vi "Configure Signaling RF UL Location A.vi"(8 "error in (no error)":errorcluster, 9 "UL Location A (Mid)":i32(ring) items=["Mid", "Low", "High", "User"], 10 "Cell Name (\"Cell Name\")":string="Cell Name", 11 "VISA resource name":refnum<visa-resource-name>) -> (0 "error out":errorcluster, 3 "VISA resource name out":refnum<visa-resource-name>)   [LabVIEW 2020, in "Rohde&Schwarz CMWXP NR FR1 Measurement.lvlib"]
doc: "Selects a method for defining the frequency of point A, for the uplink.\n\nAttribute:\nRSCMWXPNRFR1M_ATTR_SIGNALING_RF_UL_LOCATION_A\n\nRemote-control command:\n[CONFigure:]SIGNaling:NRADio:CELL:RFSettings:UL:APOint:LOCation"
uses:
  <instrlib>/Rohde&Schwarz CMWXP NR FR1 Measurement/Rohde&Schwarz CMWXP NR FR1 Measurement.lvlib
  <instrlib>/Rohde&Schwarz CMWXP NR FR1 Measurement/Private/rsidr_core.llb/rsidr_core.lvlib
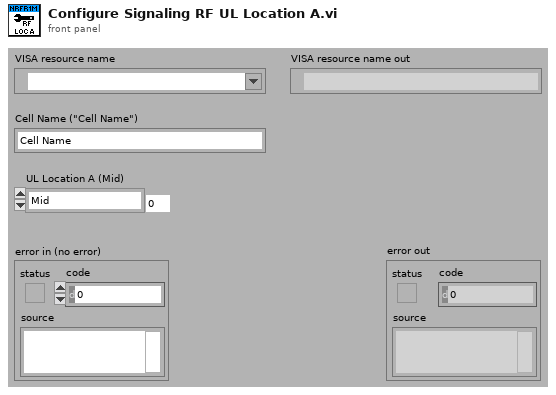
[diagram p1: front panel]
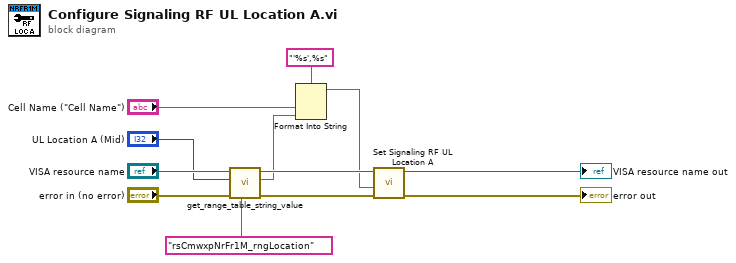
[diagram p0: block diagram]
diagram:
  n1 = call <instrlib>:"get_range_table_string_value.vi"("Range Table ID in"="rsCmwxpNrFr1M_rngLocation", "error in"="error in (no error)", "I32 input"="UL Location A (Mid)", "VISA resource name"="VISA resource name") -> ("error out"=w8:errorcluster, "String Value out"=w2:string, "VISA resource name out"=w7:refnum<visa-resource-name>)  [unwired: 5 in]
  n2 = Format Into String(format string="'%s',%s", "Cell Name (\"Cell Name\")", w2) -> (resulting string=w1:string)  [unwired: 2 in, 1 out]
  n3 = call "Set Signaling RF UL Location A"("error in (no error)"=w8, "Signaling RF UL Location A ()"=w1, "instrument handle"=w7) -> ("error out"=→"error out":errorcluster, "instrument handle out"=→"VISA resource name out":refnum<visa-resource-name>)  [unwired: 7 in]
